vi "ToolBarButtonDraw_cursor.vi"(6 "Color":u32(colorbox), 10 "rect":T1, 11 "Pict IN":picture) -> (3 "Pict OUT":picture)   [LabVIEW 2020, in "Sgraph_lib_V1.lvlib" / "Gviewer.lvclass"]
doc: "Draw Focus icon in button bar"
uses:
  Gviewer.lvclass
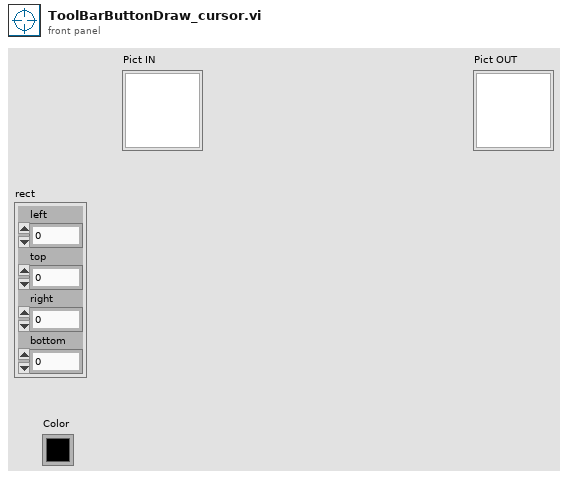
[diagram p1: front panel]
types:
  T1 = cluster{"left":i16, "top":i16, "right":i16, "bottom":i16}
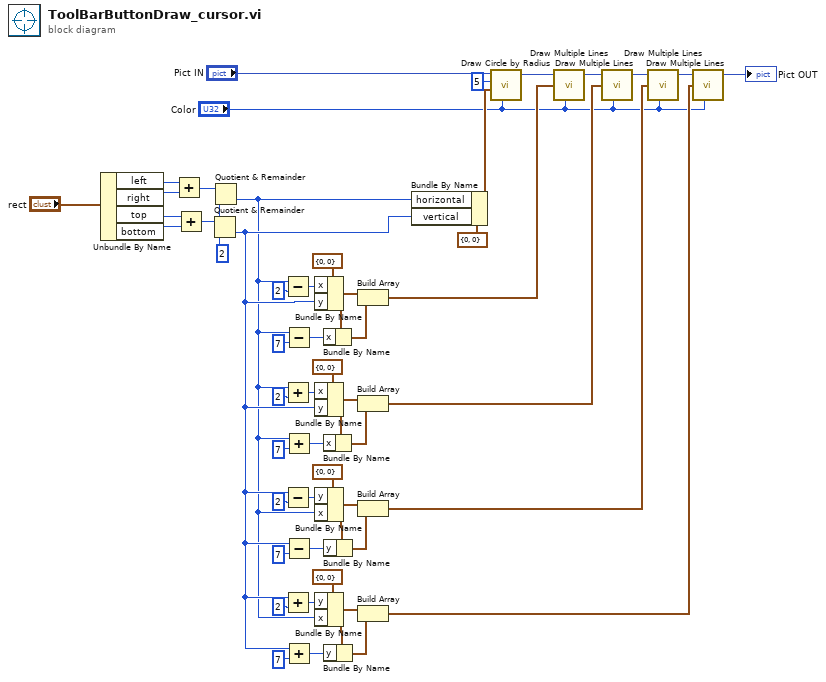
[diagram p0: block diagram]
diagram:
  w43 = i16 2 ("y")
  n1 = Unbundle By Name("rect") -> ("left"=w49:i16, "right"=w48:i16, "top"=w47:i16, "bottom"=w46:i16)
  n2 = Add(x=w49, y=w48) -> (x+y=w45:i16)
  n3 = Add(x=w47, y=w46) -> (x+y=w44:i16)
  n4 = Quotient & Remainder(x=w44, y=w43) -> (floor(x/y)=w4:i16)  [unwired: 1 out]
  n5 = Quotient & Remainder(x=w45, y=w43) -> (floor(x/y)=w3:i16)  [unwired: 1 out]
  n6 = Subtract(x=w3, y=i16 2) -> (x-y=w36:i16)
  n7 = Add(x=w3, y=i16 2) -> (x+y=w23:i16)
  n8 = Subtract(x=w4, y=i16 2) -> (x-y=w17:i16)
  n9 = Add(x=w4, y=i16 2) -> (x+y=w7:i16)
  n10 = Subtract(x=w3, y=i16 7) -> (x-y=w34:i16)
  n11 = Add(x=w3, y=i16 7) -> (x+y=w25:i16)
  n12 = Subtract(x=w4, y=i16 7) -> (x-y=w15:i16)
  n13 = Add(x=w4, y=i16 7) -> (x+y=w9:i16)
  n14 = Bundle By Name(cluster=cluster{"x":i16, "y":i16} {"x"=0, "y"=0}, "x"=w36, "y"=w4) -> (w33:cluster{"x":i16, "y":i16})
  n15 = Bundle By Name(cluster=cluster{"x":i16, "y":i16} {"x"=0, "y"=0}, "x"=w23, "y"=w4) -> (w26:cluster{"x":i16, "y":i16})
  n16 = Bundle By Name(cluster=cluster{"x":i16, "y":i16} {"x"=0, "y"=0}, "y"=w17, "x"=w3) -> (w14:cluster{"x":i16, "y":i16})
  n17 = Bundle By Name(cluster=cluster{"x":i16, "y":i16} {"x"=0, "y"=0}, "y"=w7, "x"=w3) -> (w10:cluster{"x":i16, "y":i16})
  n18 = Bundle By Name(cluster=w33, "x"=w34) -> (w32:cluster{"x":i16, "y":i16})
  n19 = Bundle By Name(cluster=w26, "x"=w25) -> (w27:cluster{"x":i16, "y":i16})
  n20 = Bundle By Name(cluster=w14, "y"=w15) -> (w13:cluster{"x":i16, "y":i16})
  n21 = Bundle By Name(cluster=w10, "y"=w9) -> (w11:cluster{"x":i16, "y":i16})
  n22 = Build Array(w33, w32) -> (w31:cluster{"x":i16, "y":i16}[])
  n23 = Build Array(w26, w27) -> (w20:cluster{"x":i16, "y":i16}[])
  n24 = Build Array(w14, w13) -> (w12:cluster{"x":i16, "y":i16}[])
  n25 = Build Array(w10, w11) -> (w2:cluster{"x":i16, "y":i16}[])
  n26 = Bundle By Name(cluster=cluster{"horizontal":i16, "vertical":i16} {"horizontal"=0, "vertical"=0} ("pixel center"), "horizontal"=w3, "vertical"=w4) -> (w50:cluster{"horizontal":i16, "vertical":i16})
  n27 = call <vilib>:"Draw Circle by Radius.vi"("color(black)"="Color", "pixel center"=w50, "radius"=i16 5, "picture"="Pict IN") -> ("new picture"=w42:picture)  [unwired: 7 in]
  n28 = call <vilib>:"Draw Multiple Lines.vi"("picture"=w42, "line endpoints"=w31, "color(black)"="Color") -> ("new picture"=w41:picture)  [unwired: 6 in]
  n29 = call <vilib>:"Draw Multiple Lines.vi"("picture"=w41, "line endpoints"=w20, "color(black)"="Color") -> ("new picture"=w40:picture)  [unwired: 6 in]
  n30 = call <vilib>:"Draw Multiple Lines.vi"("picture"=w40, "line endpoints"=w12, "color(black)"="Color") -> ("new picture"=w39:picture)  [unwired: 6 in]
  n31 = call <vilib>:"Draw Multiple Lines.vi"("picture"=w39, "line endpoints"=w2, "color(black)"="Color") -> ("new picture"=→"Pict OUT":picture)  [unwired: 6 in]
